vi "PEM Control Panel (No Objects).vi"() -> ()   [LabVIEW 2017]
panel:
  out "Ready":bool
  in  "wavelength":dbl[unit] min=0.0 max=1.99999e-05 step=1.0000000000000002e-10
  in  "Retardation 2":dbl=1.0 min=0.0 max=1.0 step=0.001
  in  "Set Retardation":bool
  in  "Set Wavelength":bool
  in  "Inhibit":bool
  out "Retardation":dbl
  out "Wavelength":dbl[unit]
  out "Frequency output":string
  out "stop":bool
  out "VISA resource name out":refnum<visa-resource-name>
  out "error out":errorcluster
  in  "VISA resource name":refnum<visa-resource-name>="COM3"
  in  "error in (no error)":errorcluster
  # "On"
  # "Off"
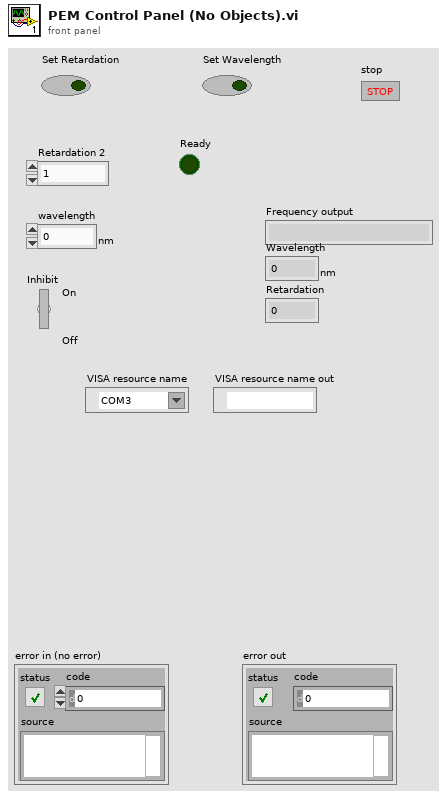
[diagram p1: front panel]
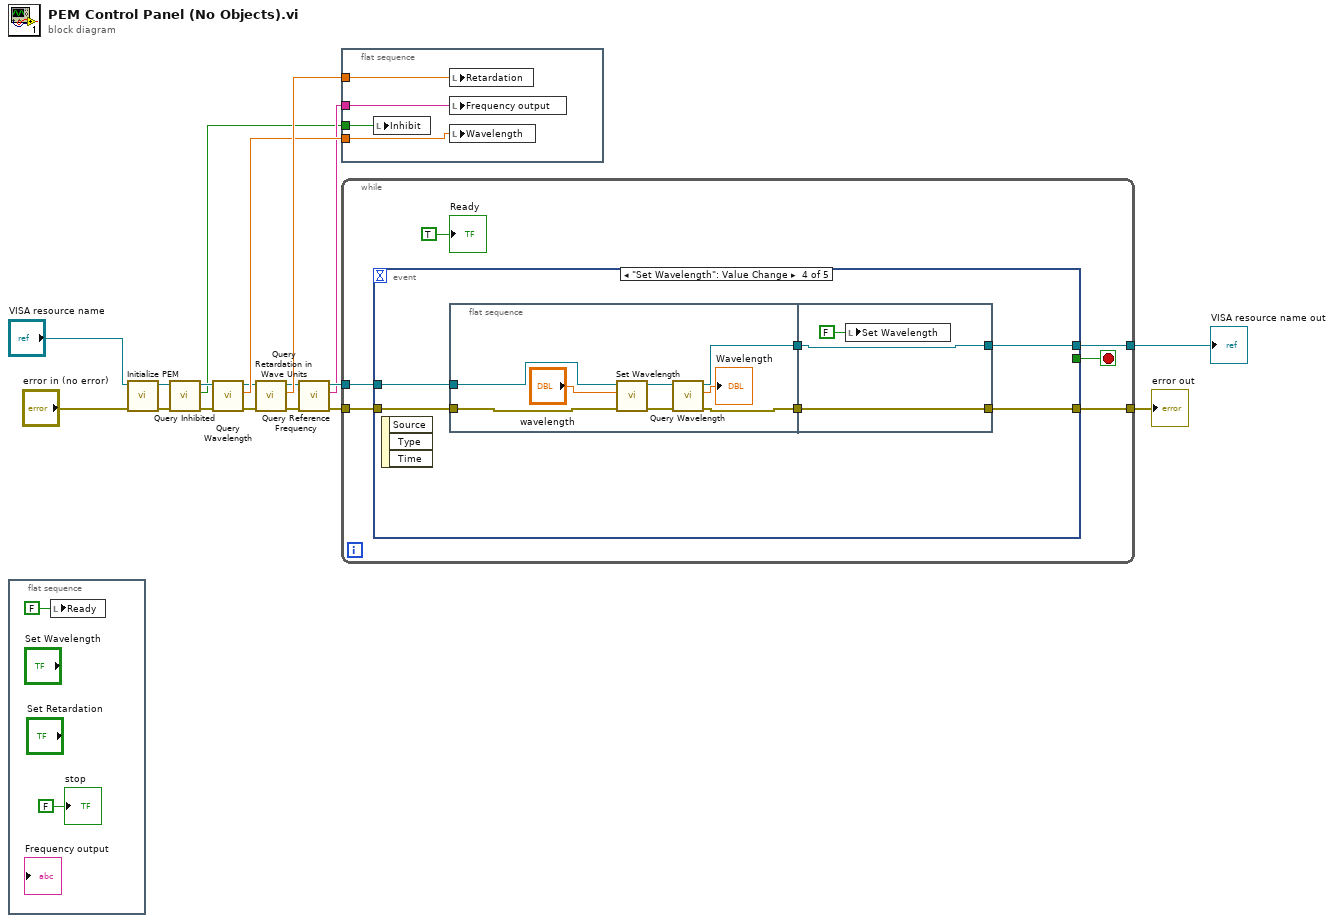
[diagram p0: block diagram]
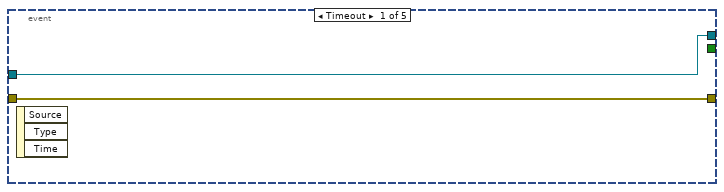
[diagram p2: hidden frame]
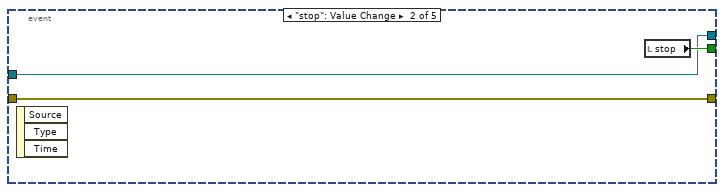
[diagram p3: hidden frame]
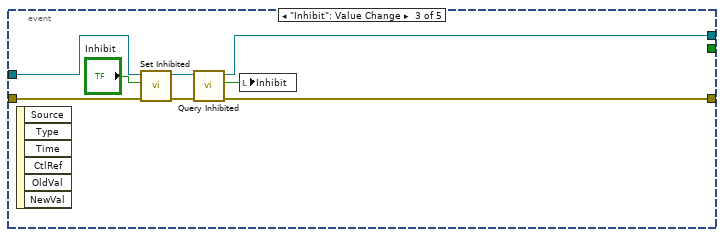
[diagram p4: hidden frame]
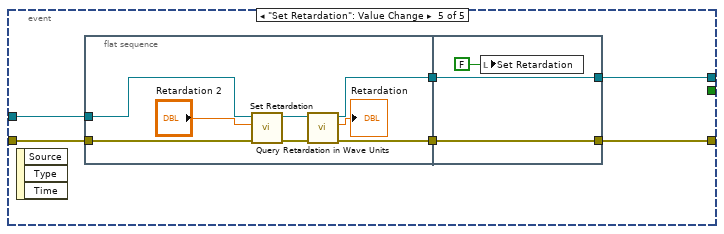
[diagram p5: hidden frame]
diagram:
  n1 = flat-sequence {
    frame #0 {
      n2 = local write "Ready"(FALSE ("Ready")) -> ()
      "stop" <- FALSE ("stop")
    }
  }
  n3 = call "Initialize PEM.vi"("error in (no error)"="error in (no error)", "VISA resource name"="VISA resource name") -> ("error out"=w5:errorcluster, "VISA resource name out"=w4:refnum<visa-resource-name>)  [unwired: 8 in]
  n4 = call "Query Inhibited.vi"("error in (no error)"=w5, "VISA resource name"=w4) -> ("error out"=w2:errorcluster, "Inibit"=w1:bool, "VISA resource name out"=w3:refnum<visa-resource-name>)  [unwired: 7 in]
  n5 = call "Query Wavelength.vi"("error in (no error)"=w2, "VISA resource name"=w3) -> ("error out"=w9:errorcluster, "Wavelength"=w11:dbl[unit], "VISA resource name out"=w8:refnum<visa-resource-name>)  [unwired: 7 in]
  n6 = call "Query Retardation in Wave Units.vi"("error in (no error)"=w9, "VISA resource name"=w8) -> ("error out"=w6:errorcluster, "Fraction of wave Retardation"=w13:dbl, "VISA resource name out"=w7:refnum<visa-resource-name>)  [unwired: 7 in]
  n7 = call "Query Reference Frequency.vi"("error in (no error)"=w6, "VISA resource name"=w7) -> ("error out"=w14:errorcluster, "Frequency output"=w10:string, "VISA resource name out"=w12:refnum<visa-resource-name>)  [unwired: 7 in]
  n8 = flat-sequence {
    tunnel: w13 -> [w24]
    tunnel: w11 -> [w22]
    tunnel: w10 -> [w23]
    tunnel: w1 -> [w21]
    frame #0 {
      n9 = local write "Inhibit"(w21) -> ()
      n10 = local write "Retardation"(w24) -> ()
      n11 = local write "Frequency output"(w23) -> ()
      n12 = local write "Wavelength"(w22) -> ()
    }
  }
  n13 = while {
    tunnel: [w30] -> w16
    tunnel: [w29] -> w15
    tunnel: w14 -> [w27]
    tunnel: w12 -> [w26]
    stop <- w28 stop-if-true
    n14 = event shown="[3] \"Set Wavelength\": Value Change" {
      selector: _ -> [_ _ _ _ _]
      dyn-events: _ -> [_ _ _ _ _]
      timeout: _ -> [_ _ _ _ _]
      tunnel: w27 -> [w32 w34 w42 w48 w66]
      tunnel: w26 -> [w31 w33 w43 w49 w65]
      tunnel: [w32 w34 w39 w46 w63] -> w30
      tunnel: [w31 w33 w38 w47 w64] -> w29
      tunnel: [_ w35 _ _ _] -> w28
      event Timeout {
        n15 = event-data() -> ()  [unwired: 1 in, 3 out]
      }
      event "stop": Value Change {
        n16 = event-data() -> ()  [unwired: 1 in, 3 out]
        n17 = local read "stop"() -> (w35:bool)
      }
      event "Inhibit": Value Change {
        n18 = event-data() -> ()  [unwired: 1 in, 6 out]
        n19 = call "Set Inhibited.vi"("error in (no error)"=w42, "Inhibit"="Inhibit", "VISA resource name"=w43) -> ("error out"=w40:errorcluster, "VISA resource name out"=w41:refnum<visa-resource-name>)  [unwired: 6 in, 1 out]
        n20 = call "Query Inhibited.vi"("error in (no error)"=w40, "VISA resource name"=w41) -> ("error out"=w39:errorcluster, "Inibit"=w37:bool, "VISA resource name out"=w38:refnum<visa-resource-name>)  [unwired: 7 in]
        n21 = local write "Inhibit"(w37) -> ()
      }
      event "Set Wavelength": Value Change {
        n22 = event-data() -> ()  [unwired: 1 in, 3 out]
        n23 = flat-sequence {
          tunnel: w49 -> [w57]
          tunnel: w48 -> [w56]
          tunnel: [w54] -> w45
          tunnel: [w53] -> w44
          tunnel: [w59] -> w46
          tunnel: [w60] -> w47
          tunnel: w45 -> [w60]
          tunnel: w44 -> [w59]
          frame #0 {
            n24 = call "Set Wavelength.vi"("error in (no error)"=w56, "wavelength"="wavelength", "VISA resource name"=w57) -> ("error out"=w51:errorcluster, "VISA resource name out"=w52:refnum<visa-resource-name>)  [unwired: 5 in, 2 out]
            n25 = call "Query Wavelength.vi"("error in (no error)"=w51, "VISA resource name"=w52) -> ("error out"=w53:errorcluster, "Wavelength"=→"Wavelength":dbl[unit], "VISA resource name out"=w54:refnum<visa-resource-name>)  [unwired: 7 in]
          }
          frame #1 {
            n26 = local write "Set Wavelength"(FALSE ("Set Wavelength")) -> ()
          }
        }
      }
      event "Set Retardation": Value Change {
        n27 = event-data() -> ()  [unwired: 1 in, 3 out]
        n28 = flat-sequence {
          tunnel: w66 -> [w73]
          tunnel: w65 -> [w72]
          tunnel: [w70] -> w62
          tunnel: [w68] -> w61
          tunnel: [w76] -> w63
          tunnel: [w77] -> w64
          tunnel: w62 -> [w77]
          tunnel: w61 -> [w76]
          frame #0 {
            n29 = call "Set Retardation.vi"("error in (no error)"=w73, "Retardation"="Retardation 2", "VISA resource name"=w72) -> ("error out"=w69:errorcluster, "VISA resource name out"=w71:refnum<visa-resource-name>)  [unwired: 6 in, 1 out]
            n30 = call "Query Retardation in Wave Units.vi"("error in (no error)"=w69, "VISA resource name"=w71) -> ("error out"=w68:errorcluster, "Fraction of wave Retardation"=→"Retardation":dbl, "VISA resource name out"=w70:refnum<visa-resource-name>)  [unwired: 7 in]
          }
          frame #1 {
            n31 = local write "Set Retardation"(FALSE ("Set Retardation")) -> ()
          }
        }
      }
    }
    "Ready" <- TRUE ("Ready")
  }
  "error out" <- w16
  "VISA resource name out" <- w15
